vi "Init LCOS Menu.vi"(0 "Menu Refnum (in)":refnum<k9>, 3 "error in (no error)":errorcluster) -> (6 "Menu Refnum (out)":refnum<k9>, 9 "error out":errorcluster)   [LabVIEW 2011]
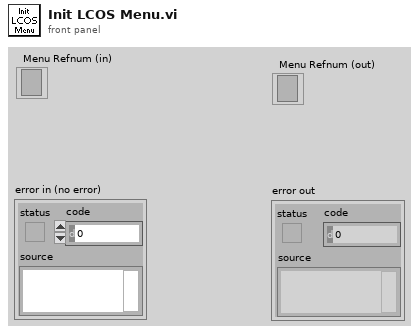
[diagram p1: front panel]
types:
  T1 = cluster{"Menu Item":string, "is submenu":bool, "short cut":cluster{"include Shift key?":bool, "shortcut key":string}, "is checked":bool, "is enabled":bool}
  T2 = cluster{"include Shift key?":bool, "shortcut key":string}[]
  T3 = cluster{"include Shift key?":bool, "include Ctrl key? ":bool, "shortcut key":string}
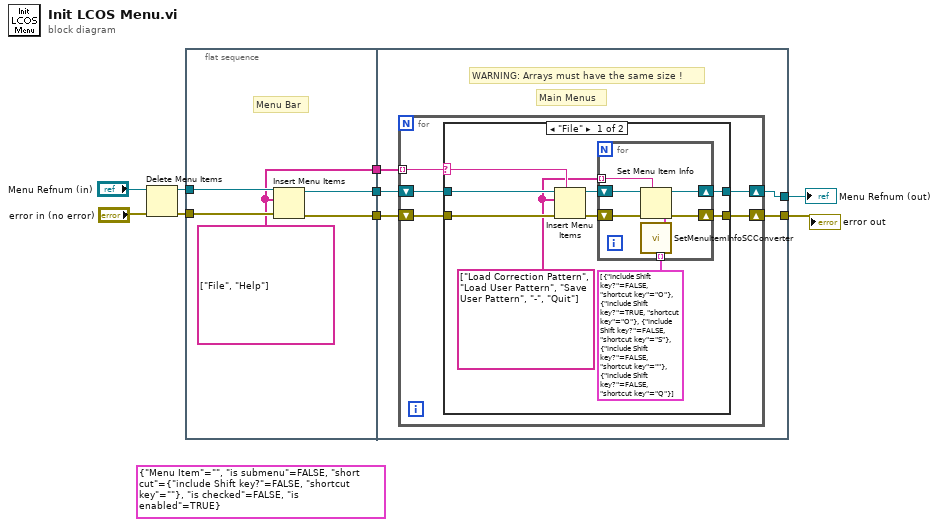
[diagram p0: block diagram]
diagram:
  (unwired) T1 {"Menu Item"="", "is submenu"=FALSE, "short cut"={"include Shift key?"=FALSE, "shortcut key"=""}, "is checked"=FALSE, "is enabled"=TRUE}
  n1 = Delete Menu Items(6:"error in (no error)", 9:"Menu Refnum (in)") -> (0:w6:errorcluster, 3:w7:refnum<k9>)  [unwired: 2 in]
  n2 = flat-sequence {
    tunnel: w7 -> [w14]
    tunnel: w6 -> [w13]
    tunnel: [w12] -> w5
    tunnel: [w11] -> w4
    tunnel: [w10] -> w3
    tunnel: w5 -> [w19]
    tunnel: w4 -> [w18]
    tunnel: w3 -> [w17]
    tunnel: [w16] -> w2
    tunnel: [w15] -> w1
    frame #0 {
      w10 = string[] ["File", "Help"] ("item names")
      # "Menu Bar"
      n3 = Insert Menu Items(6:w13, 8:w10, 9:w14) -> (0:w11:errorcluster, 3:w12:refnum<k9>)  [unwired: 3 in, 1 out]
    }
    frame #1 {
      # "WARNING: Arrays must have the same size !"
      # "Main Menus"
      n4 = for {
        shift-right: [w21] -> w16
        shift-left: w19 -> [w24]
        shift-right: [w20] -> w15
        shift-left: w18 -> [w23]
        tunnel: w17 -> [w22] mode=indexing
        n5 = case shown="\"File\"" w22 {
          selector: w22 -> [w31 _]
          tunnel: w24 -> [w33 w42]
          tunnel: w23 -> [w32 w41]
          tunnel: [w26 w42] -> w21
          tunnel: [w25 w41] -> w20
          frame "File" {
            w28 = string[] ["Load Correction Pattern", "Load User Pattern", "Save User Pattern", "-", "Quit"] ("item names")
            n6 = Insert Menu Items(5:w31, 6:w32, 8:w28, 9:w33) -> (0:w29:errorcluster, 3:w30:refnum<k9>)  [unwired: 2 in, 1 out]
            n7 = for {
              shift-right: [w37] -> w26
              shift-left: w30 -> [w40]
              shift-right: [w38] -> w25
              shift-left: w29 -> [w39]
              tunnel: w28 -> [w36] mode=indexing
              tunnel: T2 [{"include Shift key?"=FALSE, "shortcut key"="O"}, {"include Shift key?"=TRUE, "shortcut key"="O"}, {"include Shift key?"=FALSE, "shortcut key"="S"}, {"include Shift key?"=FALSE, "shortcut key"=""}, {"include Shift key?"=FALSE, "shortcut key"="Q"}] -> [w35] mode=indexing
              n8 = call <vilib>:"SetMenuItemInfoSCConverter.vi"("short cut in"=w35) -> ("short cut out"=w34:T3)
              n9 = Set Menu Item Info(4:w34, 7:w36, 8:w39, 11:w40) -> (0:w38:errorcluster, 3:w37:refnum<k9>)  [unwired: 3 in]
            }
          }
          frame "-", Default {
          }
        }
      }
    }
  }
  "Menu Refnum (out)" <- w2
  "error out" <- w1
